vi "open_browser_send_url.vi"(11 "Enter a URL and run the VI":string="www.ni.com") -> ()   [LabVIEW 2016]
doc: "This VI uses ActiveX to open IE in its own window and point it to the URL typed into the string control."
panel:
  in  "SHDocVw.IWebBrowser2":refnum<k7>
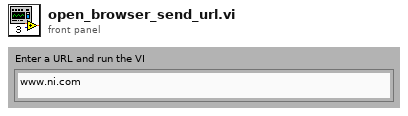
[diagram p1: front panel]
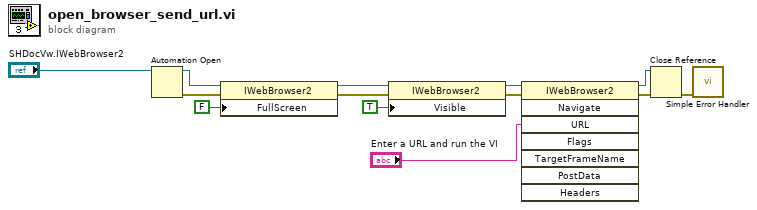
[diagram p0: block diagram]
diagram:
  n1 = Automation Open(Automation Refnum="SHDocVw.IWebBrowser2") -> (Automation Refnum=w13:refnum<k7>, error out=w12:errorcluster)  [unwired: 3 in]
  n2 = property class="IWebBrowser2"(reference=w13, error in=w12, "FullScreen"=FALSE) -> (reference out=w3:refnum<k7>, error out=w2:errorcluster)
  n3 = property class="IWebBrowser2"(reference=w3, error in=w2, "Visible"=TRUE) -> (reference out=w9:refnum<k7>, error out=w10:errorcluster)
  n4 = invoke class="IWebBrowser2" method="Navigate"(reference=w9, error in=w10, "URL"="Enter a URL and run the VI") -> (reference out=w6:refnum<k7>, error out=w7:errorcluster)  [unwired: 5 in, 6 out]
  n5 = Close Reference(reference=w6, error in (no error)=w7) -> (error out=w5:errorcluster)
  n6 = call <vilib>:"Simple Error Handler.vi"("error in (no error)"=w5) -> ()  [unwired: 4 in, 5 out]
